vi "PH_Cont-601k_PowerUnit.ProcCases.vi"(0 "i ref in":refnum<vi>, 1 "selector":string, 2 "Data":T1, 3 "call cluster":T2={"Object"="", "Selector"="", "CallType"=enum."synchronous", "Async Object"="", "Async Selector"="", "Data Descriptor"="", "Data"=[], "Error #"=0, "Expire"=0}, 5 "error in (no error)":errorcluster) -> (14 "i ref out":refnum<vi>, 17 "answer cluster":T2={"Object"="", "Selector"="", "CallType"=enum."synchronous", "Async Object"="", "Async Selector"="", "Data Descriptor"="", "Data"=[], "Error #"=0, "Expire"=0}, 19 "error out":errorcluster)   [LabVIEW 2014, in "PH_Cont-601k_PowerUnit.lvlib"]
doc: "This method is called by a process from within the default case in the event loop. The methods of a class that are linked to events will be called from THIS method. Add your code here."
uses:
  PH_Cont-601k_PowerUnit.lvlib
  CS_Core/CSSystem/CoreDefs/CoreDefs.call_type.ctl
  CS_Core/BaseProcess/BaseProcess.descriptor string definition.ctl
  CS_Core/CSSystem/CoreDefs/CoreDefs.rawDataType.ctl
  PH_Basics/PH_PowerUnit_BaseClass/PH_PowerUnit_BaseClass.SM States.ctl
  CS_Core/CSSystem/CoreLib/CoreLib.string 2 byte array.vi
  CS_Core/CSSystem/CoreLib/CoreLib.byte array 2 short.vi
  CS_Core/CSSystem/CoreLib/CoreLib.byte array 2 double.vi
  CS_Core/BaseProcess/BaseProcess.lvlib
  CS_Core/CSSystem/CoreLib/CoreLib.lvlib
  CS_Core/CAEObj/CAEObj.lvlib
  PH_Basics/PH_PSDBWriter/PH_PSDBWriter.lvlib
  PH_Devices/PH_Cont-601k_PSU/PH_Cont-601k_PSU.lvlib
  PH_Basics/PH_PowerUnit_BaseClass/PH_PowerUnit_BaseClass.lvlib
  CS_Core/BaseSM/BaseSM.lvlib
  PH_Basics/PH_Common/PH_Common.lvlib
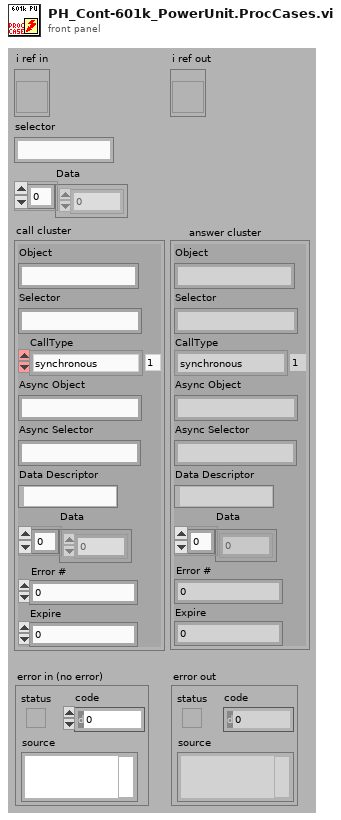
[diagram p1: front panel]
types:
  T1 = typedef "CoreDefs.rawDataType.ctl" = i8[]
  T2 = typedef "CoreDefs.call_type.ctl" = cluster{"Object":string, "Selector":string, "CallType":enum16{"simple", "synchronous", "asynchronous"}, "Async Object":string, "Async Selector":string, "Data Descriptor":T3, "Data":T1, "Error #":i32, "Expire":u32}
  T3 = typedef "BaseProcess.lvlib/BaseProcess.descriptor string definition.ctl" = string
  T4 = typedef "PH_PowerUnit_BaseClass.lvlib/PH_PowerUnit_BaseClass.SM States.ctl" = enum16{".", "Stand by", "Switch PU on", "Configure", "Set Default Voltage", "Set STANDBY", "Set READY", "Wait for Shot Cmd", "Open Dump Rods", "Open Ross Relais", "Close Ross Relais", "Switch PSU on", "Switch PSU off", "Charge", "Switch GD Channel on", "Close Dump Rods", "Rods-TO", "RR-TO", "PSU-TO", "Trigger-TO"}
  T5 = typedef "PH_PowerUnit_BaseClass.lvlib/PH_PowerUnit_BaseClass.i attribute.ctl" = cluster{"Constructor finished":bool, "PU":cluster{"In use":bool, "Service ID in use":i32, "GUI Ref":refnum<vi>}, "Enabling":cluster{"State":T6, "GUI Ref":refnum<vi>}, "Timing":cluster{"Last Shot":dbl, "Time between Shots [Sec]":dbl, "Waiting Time over?":bool, "Service ID Waiting Time":i32, "GUI Ref":refnum<vi>, "Instance":cluster{"Status":T7, "linked?":bool, "GUI Ref":refnum<vi>}}, "Sequencer":cluster{"SM State":string, "GUI Ref":refnum<vi>, "linked":bool}, "Subscribed Trendmssgs":cluster{"Tagname":string, "Status":T7, "linked?":bool, "Shot Condition":T7, "GUI Ref":refnum<vi>}[], "PP PU":T8, "Default Voltage (V)":dbl, "GUI Refs":T9, "PSDB data":cluster{"Shot Voltage [V]":dbl, "State TO SM":T4, "Write 2 early":bool}, "State TO SM":T4}
  T6 = typedef "PH_SystemInformation.lvlib/PH_SystemInformationEnabling State.ctl" = i32
  T7 = typedef "PH_StatusHandler.lvlib/PH_StatusHandler.Status.ctl" = i16
  T8 = typedef "PH_PP_Common.lvlib/PH_PP_Common.PUs.ctl" = enum16{"no Info", "PA-19mm-1", "PA-19mm-2", "PA-45mm-PILC", "PA-45mm-MAIN", "MA-PU-1", "MA-PU-2", "MA-PU-3", "MA-PU-4", "MA-PU-5", "MA-PU-6", "MA-FR", "MA-PILC", "PA-45mm-DP"}
  T9 = typedef "PH_PowerUnit_BaseClass.lvlib/PH_PowerUnit_BaseClass.GUI Refs.ctl" = cluster{"Delete Inst":refnum<vi>, "State TO SM":refnum<vi>, "State SM":refnum<vi>, "Fire":refnum<vi>}
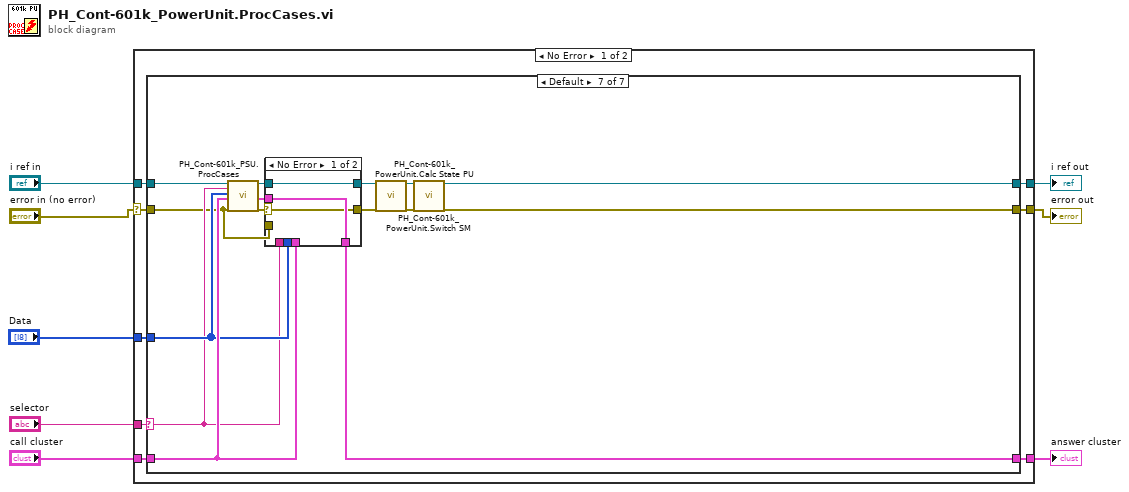
[diagram p0: block diagram]
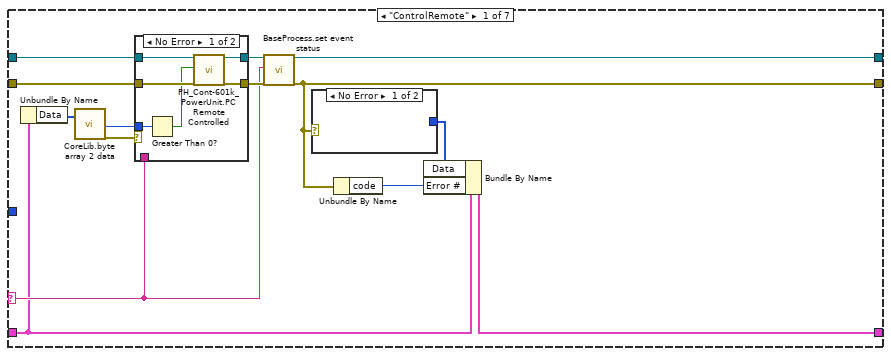
[diagram p2: hidden frame]
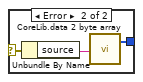
[diagram p3: hidden frame]
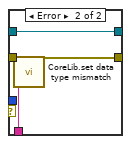
[diagram p4: hidden frame]
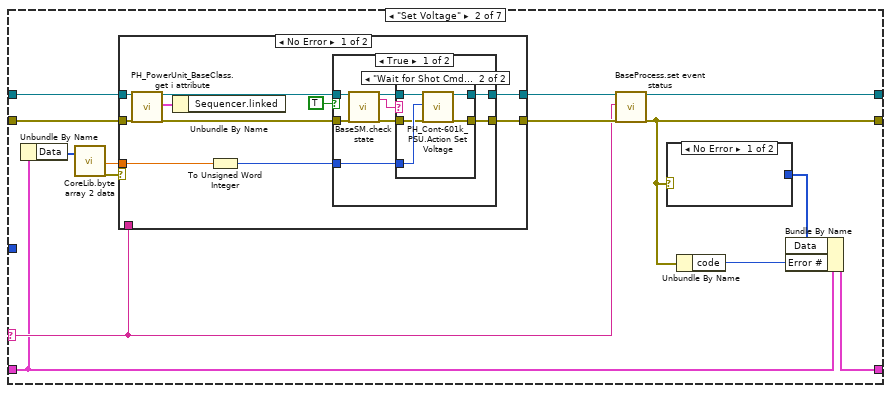
[diagram p5: hidden frame]
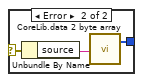
[diagram p6: hidden frame]
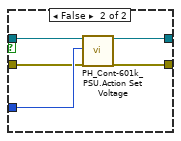
[diagram p8: hidden frame]
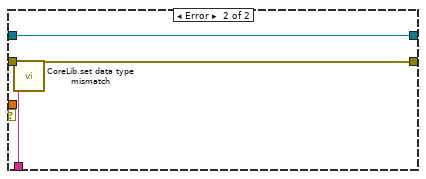
[diagram p9: hidden frame]
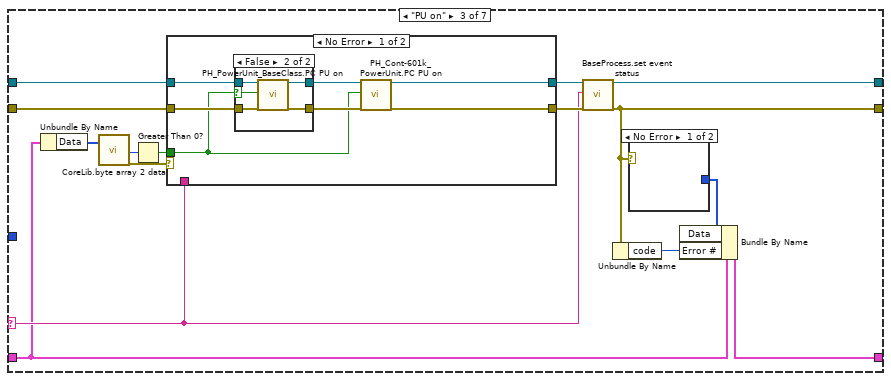
[diagram p10: hidden frame]
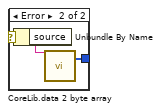
[diagram p11: hidden frame]
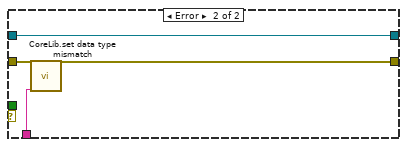
[diagram p13: hidden frame]
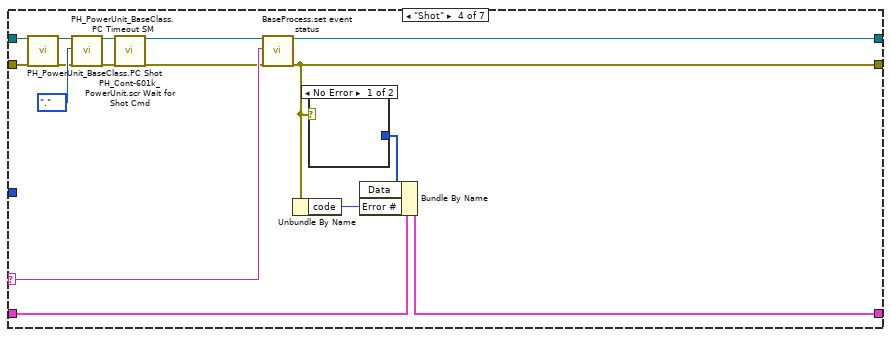
[diagram p14: hidden frame]
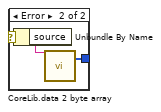
[diagram p15: hidden frame]
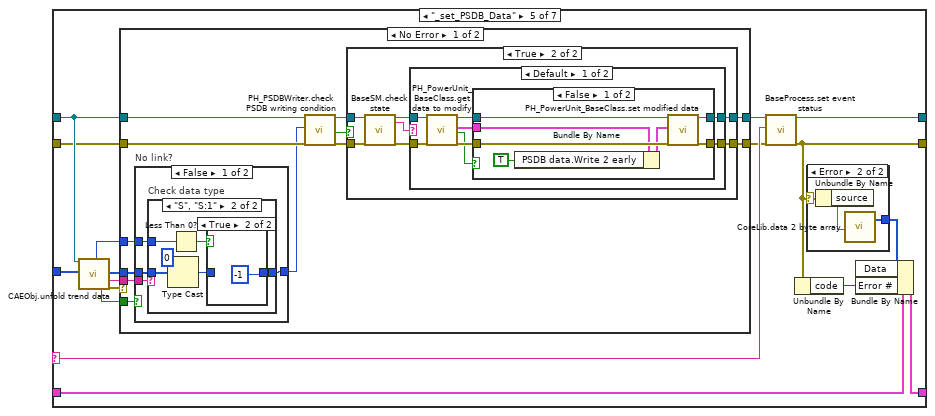
[diagram p16: hidden frame]
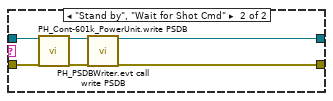
[diagram p19: hidden frame]
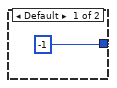
[diagram p20: hidden frame]
diagram:
  n1 = case shown="No Error" "error in (no error)" {
    selector: "error in (no error)" -> [w9 w316]
    tunnel: "selector" -> [w16 _]
    tunnel: [w15 w315] -> w7
    tunnel: "call cluster" -> [w14 w315]
    tunnel: "i ref in" -> [w13 w317]
    tunnel: [w12 w317] -> w4
    tunnel: [w11 w316] -> w3
    tunnel: "Data" -> [w10 _]
    frame No Error {
      n2 = case shown="Default" w16 {
        selector: w16 -> [w19 w46 w101 w142 w160 w241 w299]
        tunnel: w13 -> [w30 w57 w109 w138 w153 w234 w290]
        tunnel: [w21 w48 w103 w144 w164 w245 w291] -> w12
        tunnel: w14 -> [w18 w45 w100 w141 w162 w243 w301]
        tunnel: [w17 w44 w99 w140 w161 w242 w303] -> w15
        tunnel: w9 -> [w29 w56 w108 w136 w152 w233 w289]
        tunnel: [w20 w47 w102 w143 w163 w244 w292] -> w11
        tunnel: w10 -> [_ _ _ _ w154 w235 w300]
        frame "ControlRemote" {
          n3 = Unbundle By Name(w18) -> ("Data"=w28:T1)
          n4 = call-poly "CoreLib.byte array 2 data.vi"("byteArray"=w28) -> ("i16"=w26:i16, "error out"=w27:errorcluster)  [unwired: 16 in, 1 out]
          n5 = case shown="No Error" w27 {
            tunnel: [w36 w43] -> w22
            tunnel: w30 -> [w39 w43]
            tunnel: w29 -> [w38 w42]
            tunnel: [w35 w41] -> w23
            tunnel: w19 -> [_ w40]
            tunnel: w26 -> [w37 _]
            frame No Error {
              n6 = Greater Than 0?(x=w37) -> (x > 0?=w34:bool)
              n7 = call "PH_Cont-601k_PowerUnit.PC Remote Controlled.vi"("VI in"=w39, "RC controlled?"=w34, "error in (no error)"=w38) -> ("VI out"=w36:refnum<vi>, "error out"=w35:errorcluster)  [unwired: 15 in]
            }
            frame Error {
              n8 = call "CoreLib.set data type mismatch.vi"("error in (no error)"=w42, "error source"=w40) -> ("error out"=w41:errorcluster)  [unwired: 17 in]
            }
          }
          n9 = call "BaseProcess.set event status.vi"("i ref in"=w22, "EventStatus"=w19, "error in (no error)"=w23) -> ("i ref out"=w21:refnum<vi>, "error out"=w20:errorcluster)  [unwired: 14 in, 1 out]
          n10 = case shown="No Error" w20 {
            selector: w20 -> [_ w33]
            tunnel: [_ w31] -> w24
            frame No Error {
            }
            frame Error {
              n11 = Unbundle By Name(w33) -> ("source"=w32:string)
              n12 = call-poly "CoreLib.data 2 byte array.vi"("string"=w32) -> ("byteArray out"=w31:T1)  [unwired: 18 in]
            }
          }
          n13 = Unbundle By Name(w20) -> ("code"=w25:i32)
          n14 = Bundle By Name(cluster=w18, "Data"=w24, "Error #"=w25) -> (w17:T2)
        }
        frame "Set Voltage" {
          n15 = Unbundle By Name(w45) -> ("Data"=w55:T1)
          n16 = call-poly "CoreLib.byte array 2 data.vi"("byteArray"=w55) -> ("d64"=w53:dbl, "error out"=w54:errorcluster)  [unwired: 16 in, 1 out]
          n17 = case shown="No Error" w54 {
            tunnel: [w69 w94] -> w49
            tunnel: w57 -> [w65 w94]
            tunnel: w56 -> [w66 w93]
            tunnel: [w70 w92] -> w50
            tunnel: w46 -> [_ w91]
            tunnel: w53 -> [w68 _]
            frame No Error {
              n18 = call "PH_PowerUnit_BaseClass.get i attribute.vi"("i ref in"=w65, "error in (no error)"=w66) -> ("i ref out"=w64:refnum<vi>, "i attribute"=w62:T5, "error out"=w63:errorcluster)  [unwired: 15 in]
              n19 = Unbundle By Name(w62) -> ()  [unwired: 1 out]
              n20 = To Unsigned Word Integer(number=w68) -> (unsigned 16bit integer=w67:u16)
              n21 = case shown="True" TRUE {
                tunnel: [w78 w90] -> w70
                tunnel: [w77 w89] -> w69
                tunnel: w67 -> [w76 w88]
                tunnel: w64 -> [w72 w87]
                tunnel: w63 -> [w71 w86]
                frame True {
                  n22 = call "BaseSM.check state.vi"("i ref in"=w72, "error in (no error)"=w71) -> ("i ref out"=w75:refnum<vi>, "actualState"=w73:string, "error out"=w74:errorcluster)  [unwired: 12 in, 3 out]
                  n23 = case shown="\"Wait for Shot Cmd\"" w73 {
                    tunnel: [w79 w85] -> w78
                    tunnel: [w80 w84] -> w77
                    tunnel: w76 -> [_ w83]
                    tunnel: w75 -> [w80 w82]
                    tunnel: w74 -> [w79 w81]
                    frame Default {
                    }
                    frame "Wait for Shot Cmd" {
                      n24 = call "PH_Cont-601k_PSU.Action Set Voltage.vi"("VI in"=w82, "Voltage [V]"=w83, "error in (no error)"=w81) -> ("VI out"=w84:refnum<vi>, "error out"=w85:errorcluster)  [unwired: 15 in]
                    }
                  }
                }
                frame False {
                  n25 = call "PH_Cont-601k_PSU.Action Set Voltage.vi"("VI in"=w87, "Voltage [V]"=w88, "error in (no error)"=w86) -> ("VI out"=w89:refnum<vi>, "error out"=w90:errorcluster)  [unwired: 15 in]
                }
              }
            }
            frame Error {
              n26 = call "CoreLib.set data type mismatch.vi"("error in (no error)"=w93, "error source"=w91) -> ("error out"=w92:errorcluster)  [unwired: 17 in]
            }
          }
          n27 = call "BaseProcess.set event status.vi"("i ref in"=w49, "EventStatus"=w46, "error in (no error)"=w50) -> ("i ref out"=w48:refnum<vi>, "error out"=w47:errorcluster)  [unwired: 14 in, 1 out]
          n28 = case shown="No Error" w47 {
            selector: w47 -> [_ w60]
            tunnel: [_ w58] -> w51
            frame No Error {
            }
            frame Error {
              n29 = Unbundle By Name(w60) -> ("source"=w59:string)
              n30 = call-poly "CoreLib.data 2 byte array.vi"("string"=w59) -> ("byteArray out"=w58:T1)  [unwired: 18 in]
            }
          }
          n31 = Unbundle By Name(w47) -> ("code"=w52:i32)
          n32 = Bundle By Name(cluster=w45, "Data"=w51, "Error #"=w52) -> (w44:T2)
        }
        frame "PU on" {
          n33 = Unbundle By Name(w100) -> ("Data"=w98:T1)
          n34 = call-poly "CoreLib.byte array 2 data.vi"("byteArray"=w98) -> ("i16"=w97:i16, "error out"=w95:errorcluster)  [unwired: 16 in, 1 out]
          n35 = Greater Than 0?(x=w97) -> (x > 0?=w96:bool)
          n36 = case shown="No Error" w95 {
            tunnel: w109 -> [w115 w128]
            tunnel: [w118 w128] -> w104
            tunnel: w108 -> [w119 w130]
            tunnel: [w117 w129] -> w105
            tunnel: w101 -> [_ w127]
            tunnel: w96 -> [w113 _]
            frame No Error {
              n37 = case shown="False" w113 {
                selector: w113 -> [_ w122]
                tunnel: w119 -> [w120 w126]
                tunnel: [w120 w125] -> w116
                tunnel: w115 -> [w121 w124]
                tunnel: [w121 w123] -> w114
                frame True {
                }
                frame False {
                  n38 = call "PH_PowerUnit_BaseClass.PC PU on.vi"("i ref in"=w124, "PU on"=w122, "error in (no error)"=w126) -> ("i ref out"=w123:refnum<vi>, "error out"=w125:errorcluster)  [unwired: 15 in]
                }
              }
              n39 = call "PH_Cont-601k_PowerUnit.PC PU on.vi"("i ref in"=w114, "PU on"=w113, "error in (no error)"=w116) -> ("i ref out"=w118:refnum<vi>, "error out"=w117:errorcluster)  [unwired: 15 in]
            }
            frame Error {
              n40 = call "CoreLib.set data type mismatch.vi"("error in (no error)"=w130, "error source"=w127) -> ("error out"=w129:errorcluster)  [unwired: 17 in]
            }
          }
          n41 = call "BaseProcess.set event status.vi"("i ref in"=w104, "EventStatus"=w101, "error in (no error)"=w105) -> ("i ref out"=w103:refnum<vi>, "error out"=w102:errorcluster)  [unwired: 14 in, 1 out]
          n42 = Unbundle By Name(w102) -> ("code"=w107:i32)
          n43 = case shown="No Error" w102 {
            selector: w102 -> [_ w112]
            tunnel: [_ w110] -> w106
            frame No Error {
            }
            frame Error {
              n44 = Unbundle By Name(w112) -> ("source"=w111:string)
              n45 = call-poly "CoreLib.data 2 byte array.vi"("string"=w111) -> ("byteArray out"=w110:T1)  [unwired: 18 in]
            }
          }
          n46 = Bundle By Name(cluster=w100, "Data"=w106, "Error #"=w107) -> (w99:T2)
        }
        frame "Shot" {
          n47 = call "PH_PowerUnit_BaseClass.PC Shot.vi"("i ref in"=w138, "error in (no error)"=w136) -> ("i ref out"=w137:refnum<vi>, "error out"=w135:errorcluster)  [unwired: 16 in]
          n48 = call "PH_PowerUnit_BaseClass.PC Timeout SM.vi"("VI in"=w137, "Timeout SM"=PH_PowerUnit_BaseClass.SM_States.".", "error in (no error)"=w135) -> ("VI out"=w134:refnum<vi>, "error out"=w132:errorcluster)  [unwired: 15 in]
          n49 = call "PH_Cont-601k_PowerUnit.scr Wait for Shot Cmd.vi"("VI in"=w134, "error in (no error)"=w132) -> ("VI out"=w133:refnum<vi>, "error out"=w131:errorcluster)  [unwired: 16 in]
          n50 = call "BaseProcess.set event status.vi"("i ref in"=w133, "EventStatus"=w142, "error in (no error)"=w131) -> ("i ref out"=w144:refnum<vi>, "error out"=w143:errorcluster)  [unwired: 14 in, 1 out]
          n51 = Unbundle By Name(w143) -> ("code"=w146:i32)
          n52 = case shown="No Error" w143 {
            selector: w143 -> [_ w149]
            tunnel: [_ w147] -> w145
            frame No Error {
            }
            frame Error {
              n53 = Unbundle By Name(w149) -> ("source"=w148:string)
              n54 = call-poly "CoreLib.data 2 byte array.vi"("string"=w148) -> ("byteArray out"=w147:T1)  [unwired: 18 in]
            }
          }
          n55 = Bundle By Name(cluster=w141, "Data"=w145, "Error #"=w146) -> (w140:T2)
        }
        frame "_set_PSDB_Data" {
          n56 = call "CAEObj.unfold trend data.vi"("i ref in"=w153, "raw trend data"=w154) -> ("quality"=w155:i32, "no link"=w158:bool, "data"=w156:i8[], "typeDescriptor"=w157:string, "error out"=w159:errorcluster)  [unwired: 9 in, 4 out]
          n57 = case shown="No Error" w159 {
            tunnel: w152 -> [w170 w227]
            tunnel: [w178 w226] -> w151
            tunnel: [w177 w227] -> w150
            tunnel: w153 -> [w176 w226]
            tunnel: w158 -> [w175 _]
            tunnel: w157 -> [w174 _]
            tunnel: w156 -> [w173 _]
            tunnel: w155 -> [w172 _]
            frame No Error {
              n58 = case "No link?" shown="False" w175 {
                tunnel: [w214 -1] -> w167
                tunnel: w172 -> [w213 _]
                tunnel: w173 -> [w212 _]
                tunnel: w174 -> [w211 _]
                frame False {
                  n59 = case "Check data type" shown="\"S\", \"S:1\"" w211 {
                    tunnel: [-1 w221] -> w214
                    tunnel: w213 -> [_ w219]
                    tunnel: w212 -> [_ w217]
                    frame Default {
                    }
                    frame "S", "S:1" {
                      n60 = Type Cast(type=i16 0, x=w217) -> (*(type *) &x=w216:i16)
                      n61 = Less Than 0?(x=w219) -> (x < 0?=w220:bool)
                      n62 = case shown="True" w220 {
                        tunnel: [w222 -1] -> w221
                        tunnel: w216 -> [w223 _]
                        frame False {
                          n63 = To Long Integer(number=w223) -> (32bit integer=w222:i32)
                        }
                        frame True {
                        }
                      }
                    }
                  }
                }
                frame True {
                }
              }
              n64 = call "PH_PSDBWriter.check PSDB writing condition.vi"("i ref in"=w176, "wanted Subsystem"=w167, "error IO"=w170) -> ("i ref out"=w171:refnum<vi>, "write PSDB?"=w168:bool, "error out"=w169:errorcluster)  [unwired: 14 in]
              n65 = case shown="True" w168 {
                tunnel: w169 -> [w179 w183]
                tunnel: [w180 w186] -> w178
                tunnel: [w179 w187] -> w177
                tunnel: w171 -> [w180 w185]
                frame False {
                }
                frame True {
                  n66 = call "BaseSM.check state.vi"("i ref in"=w185, "error in (no error)"=w183) -> ("i ref out"=w184:refnum<vi>, "actualState"=w181:string, "error out"=w182:errorcluster)  [unwired: 12 in, 3 out]
                  n67 = case shown="Default" w181 {
                    tunnel: [w188 w210] -> w187
                    tunnel: [w189 w209] -> w186
                    tunnel: w184 -> [w191 w206]
                    tunnel: w182 -> [w190 w205]
                    frame Default {
                      n68 = call "PH_PowerUnit_BaseClass.get data to modify.vi"("i ref in"=w191, "error in (no error)"=w190) -> ("i ref out"=w194:refnum<vi>, "i attribute"=w192:T5, "timed out"=w193:bool, "error out"=w195:errorcluster)  [unwired: 14 in]
                      n69 = case shown="False" w193 {
                        tunnel: w195 -> [w202 w203]
                        tunnel: w194 -> [w201 w204]
                        tunnel: [w200 w204] -> w189
                        tunnel: [w199 w203] -> w188
                        tunnel: w192 -> [w198 _]
                        frame False {
                          n70 = Bundle By Name(cluster=w198, "PSDB data.Write 2 early"=TRUE) -> (w197:T5)
                          n71 = call "PH_PowerUnit_BaseClass.set modified data.vi"("i ref in"=w201, "i attribute"=w197, "error in (no error)"=w202) -> ("i ref out"=w200:refnum<vi>, "error out"=w199:errorcluster)  [unwired: 15 in]
                        }
                        frame True {
                        }
                      }
                    }
                    frame "Stand by", "Wait for Shot Cmd" {
                      n72 = call "PH_Cont-601k_PowerUnit.write PSDB.vi"("i ref in"=w206, "error IO"=w205) -> ("i ref out"=w207:refnum<vi>, "error out"=w208:errorcluster)  [unwired: 16 in]
                      n73 = call "PH_PSDBWriter.evt call write PSDB.vi"("i ref in"=w207, "error in (no error)"=w208) -> ("i ref out"=w209:refnum<vi>, "error out"=w210:errorcluster)  [unwired: 16 in]
                    }
                  }
                }
              }
            }
            frame Error {
            }
          }
          n74 = call "BaseProcess.set event status.vi"("i ref in"=w151, "EventStatus"=w160, "error in (no error)"=w150) -> ("i ref out"=w164:refnum<vi>, "error out"=w163:errorcluster)  [unwired: 14 in, 1 out]
          n75 = Unbundle By Name(w163) -> ("code"=w166:i32)
          n76 = case shown="Error" w163 {
            selector: w163 -> [_ w230]
            tunnel: [_ w228] -> w165
            frame No Error {
            }
            frame Error {
              n77 = Unbundle By Name(w230) -> ("source"=w229:string)
              n78 = call-poly "CoreLib.data 2 byte array.vi"("string"=w229) -> ("byteArray out"=w228:T1)  [unwired: 18 in]
            }
          }
          n79 = Bundle By Name(cluster=w162, "Data"=w165, "Error #"=w166) -> (w161:T2)
        }
        frame "_SMStateSequencer" {
          n80 = call "CAEObj.unfold trend data.vi"("i ref in"=w234, "raw trend data"=w235) -> ("quality"=w236:i32, "no link"=w239:bool, "data"=w237:i8[], "typeDescriptor"=w238:string, "error out"=w240:errorcluster)  [unwired: 9 in, 4 out]
          n81 = case shown="No Error" w240 {
            tunnel: w233 -> [w261 w285]
            tunnel: [w250 w284] -> w232
            tunnel: [w249 w285] -> w231
            tunnel: w234 -> [w262 w284]
            tunnel: w239 -> [w258 _]
            tunnel: w238 -> [w259 _]
            tunnel: w237 -> [w260 _]
            tunnel: w236 -> [w257 _]
            frame No Error {
              n82 = call "PH_DIM.get String.vi"("no link"=w258, "typeDescriptor"=w259, "data"=w260, "quality"=w257) -> ("Output String"=w263:string)
              n83 = call "PH_PowerUnit_BaseClass.PC Seq SM.vi"("i ref in"=w262, "SM State"=w263, "no link"=w258, "error in"=w261) -> ("i ref out"=w252:refnum<vi>, "error out"=w251:errorcluster)  [unwired: 14 in]
              n84 = call "PH_PowerUnit_BaseClass.get i attribute.vi"("i ref in"=w252, "error in (no error)"=w251) -> ("i ref out"=w254:refnum<vi>, "i attribute"=w256:T5, "error out"=w253:errorcluster)  [unwired: 15 in]
              n85 = Unbundle By Name(w256) -> ("Sequencer.SM State"=w255:string, "State TO SM"=w248:T4)
              n86 = case shown="\"Start PPPA\"" w255 {
                tunnel: w253 -> [w264 w267 w281]
                tunnel: [w264 w270 w282] -> w249
                tunnel: w254 -> [w265 w268 w279]
                tunnel: [w265 w269 w283] -> w250
                tunnel: w248 -> [_ w266 _]
                frame Default {
                }
                frame "Start Slow Devices" {
                  n87 = case shown="Default" w266 {
                    tunnel: [w271 w276] -> w270
                    tunnel: [w272 w277] -> w269
                    tunnel: w268 -> [w272 w275]
                    tunnel: w267 -> [w271 w274]
                    frame "." {
                    }
                    frame Default {
                      n88 = call "PH_PowerUnit_BaseClass.PC Timeout SM.vi"("VI in"=w275, "Timeout SM"=PH_PowerUnit_BaseClass.SM_States.".", "error in (no error)"=w274) -> ("VI out"=w277:refnum<vi>, "error out"=w276:errorcluster)  [unwired: 15 in]
                    }
                  }
                }
                frame "Start PPPA" {
                  n89 = call "PH_PowerUnit_BaseClass.PC Shot.vi"("i ref in"=w279, "error in (no error)"=w281) -> ("i ref out"=w278:refnum<vi>, "error out"=w280:errorcluster)  [unwired: 16 in]
                  n90 = call "PH_Cont-601k_PowerUnit.scr Wait for Shot Cmd.vi"("VI in"=w278, "error in (no error)"=w280) -> ("VI out"=w283:refnum<vi>, "error out"=w282:errorcluster)  [unwired: 16 in]
                }
              }
            }
            frame Error {
            }
          }
          n91 = call "BaseProcess.set event status.vi"("i ref in"=w232, "EventStatus"=w241, "error in (no error)"=w231) -> ("i ref out"=w245:refnum<vi>, "error out"=w244:errorcluster)  [unwired: 14 in, 1 out]
          n92 = Unbundle By Name(w244) -> ("code"=w247:i32)
          n93 = case shown="Error" w244 {
            selector: w244 -> [_ w288]
            tunnel: [_ w286] -> w246
            frame No Error {
            }
            frame Error {
              n94 = Unbundle By Name(w288) -> ("source"=w287:string)
              n95 = call-poly "CoreLib.data 2 byte array.vi"("string"=w287) -> ("byteArray out"=w286:T1)  [unwired: 18 in]
            }
          }
          n96 = Bundle By Name(cluster=w243, "Data"=w246, "Error #"=w247) -> (w242:T2)
        }
        frame Default {
          n97 = call "PH_Cont-601k_PSU.ProcCases.vi"("i ref in"=w290, "selector"=w299, "Data"=w300, "call cluster"=w301, "error in (no error)"=w289) -> ("i ref out"=w302:refnum<vi>, "answer cluster"=w297:T2, "error out"=w298:errorcluster)  [unwired: 12 in]
          n98 = case shown="No Error" w298 {
            selector: w298 -> [w304 _]
            tunnel: [w305 w314] -> w295
            tunnel: [w304 w313] -> w293
            tunnel: [w306 w312] -> w303
            tunnel: w302 -> [w305 w311]
            tunnel: w301 -> [_ w310]
            tunnel: w300 -> [_ w309]
            tunnel: w299 -> [_ w308]
            tunnel: w297 -> [w306 _]
            tunnel: w289 -> [_ w307]
            frame No Error {
            }
            frame Error {
              n99 = call "PH_PowerUnit_BaseClass.ProcCases.vi"("i ref in"=w311, "selector"=w308, "Data"=w309, "call cluster"=w310, "error in (no error)"=w307) -> ("i ref out"=w314:refnum<vi>, "answer cluster"=w312:T2, "error out"=w313:errorcluster)  [unwired: 12 in]
            }
          }
          n100 = call "PH_Cont-601k_PowerUnit.Calc State PU.vi"("i ref in"=w295, "error in (no error)"=w293) -> ("i ref out"=w296:refnum<vi>, "error out"=w294:errorcluster)  [unwired: 16 in]
          n101 = call "PH_Cont-601k_PowerUnit.Switch SM.vi"("VI in"=w296, "error in (no error)"=w294) -> ("VI out"=w291:refnum<vi>, "error out"=w292:errorcluster)  [unwired: 16 in]
        }
      }
    }
    frame Error {
    }
  }
  "answer cluster" <- w7
  "i ref out" <- w4
  "error out" <- w3
